vi "GetSpeed.vi"(9 "pulse positions":T2, 10 "channel":T3, 11 "Map":T1) -> (2 "pulse position data":dbl[](array[numeric]), 3 "speed (RPM)":dbl)   [LabVIEW 2017, in "AnalysisHelper.lvlib"]
uses:
  <vilib>/addons/InsightCM/Utilities/Analysis/Shared/AnalysisHelper.lvlib
  <vilib>/addons/InsightCM/Utilities/Analysis/Shared/controls/Channel.ctl
  <vilib>/addons/InsightCM/Utilities/Analysis/Shared/controls/SpeedType.ctl
  <vilib>/addons/InsightCM/Utilities/Analysis/Shared/controls/Feature.ctl
  <vilib>/addons/InsightCM/Utilities/Analysis/Shared/controls/AmplitudeScale.ctl
  <vilib>/addons/InsightCM/Utilities/Analysis/Shared/controls/PulsePositions.ctl
  <vilib>/addons/PointValueMap/controls/PointMap.ctl
  <vilib>/addons/PointValueMap/subVIs/Point_Read_double.vi
  <vilib>/addons/PointValueMap/PointValueMap.lvlib
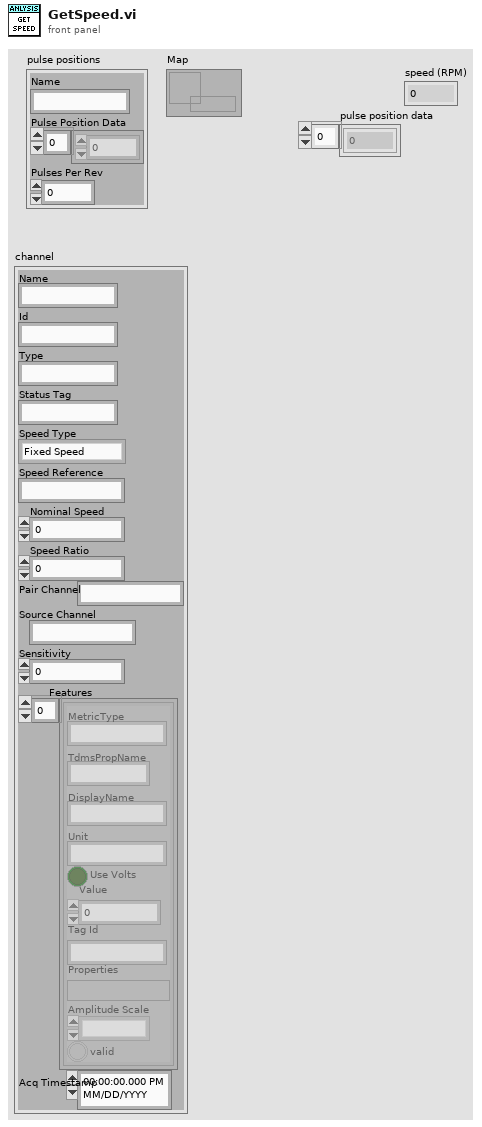
[diagram p1: front panel]
types:
  T1 = typedef "PointValueMap.lvlib/PointMap.ctl" = refnum<data-value>
  T2 = typedef "AnalysisHelper.lvlib/PulsePositions.ctl" = cluster{"Name":string, "Pulse Position Data":dbl[], "Pulses Per Rev":i32}
  T3 = typedef "AnalysisHelper.lvlib/Channel.ctl" = cluster{"Name":string, "Id":string, "Type":string, "Status Tag":string, "Speed Type":T4, "Speed Reference":string, "Nominal Speed":dbl, "Speed Ratio":dbl, "Pair Channel":string, "Source Channel":string, "Sensitivity":dbl, "Features":T5[], "Acq Timestamp":timestamp}
  T4 = typedef "AnalysisHelper.lvlib/SpeedType.ctl" = enum16{"Fixed Speed", "Tachometer", "From Map"}
  T5 = typedef "AnalysisHelper.lvlib/Feature.ctl" = cluster{"MetricType":string, "TdmsPropName":string, "DisplayName":string, "Unit":string, "Use Volts":bool, "Value":dbl, "Tag Id":string, "Properties":variant, "Amplitude Scale":T6, "valid":bool}
  T6 = typedef "AnalysisHelper.lvlib/AmplitudeScale.ctl" = enum16{"rms", "peak", "pk-pk"}
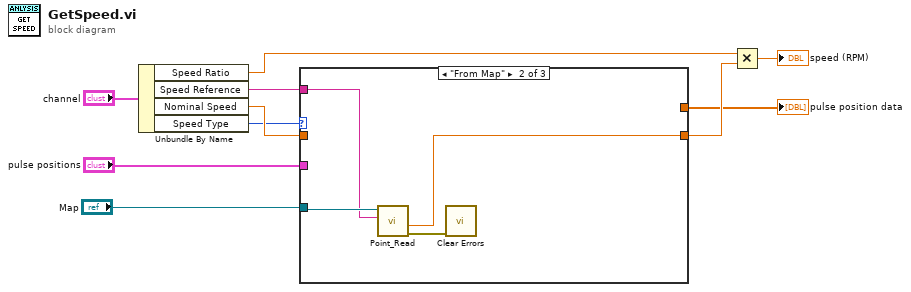
[diagram p0: block diagram]
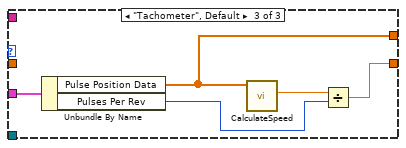
[diagram p3: hidden frame]
diagram:
  n1 = Unbundle By Name("channel") -> ("Speed Ratio"=w5:dbl, "Speed Reference"=w1:string, "Nominal Speed"=w6:dbl, "Speed Type"=w2:T4)
  n2 = case shown="\"From Map\"" w2 {
    tunnel: [w11 w13 w16] -> w7
    tunnel: "pulse positions" -> [_ _ w20]
    tunnel: w6 -> [w11 _ _]
    tunnel: [_ _ w19] -> w4
    tunnel: "Map" -> [_ w15 _]
    tunnel: w1 -> [_ w14 _]
    frame "Fixed Speed" {
    }
    frame "From Map" {
      n3 = call-poly <vilib>:"Point_Read.vi"("Tag"=w14, "Map"=w15) -> ("Error Out"=w12:errorcluster, "Value"=w13:dbl)  [unwired: 4 in, 4 out]
      n4 = call <vilib>:"Clear Errors.vi"("error in (no error)"=w12) -> ()  [unwired: 5 in, 2 out]
    }
    frame "Tachometer", Default {
      n5 = Unbundle By Name(w20) -> ("Pulse Position Data"=w19:dbl[], "Pulses Per Rev"=w17:i32)
      n6 = call <vilib>:"CalculateSpeed.vi"("Pulse Positions"=w19) -> ("Speed (RPM)"=w18:dbl)  [unwired: 9 in, 1 out]
      n7 = Divide(x=w18, y=w17) -> (x/y=w16:dbl)
    }
  }
  "pulse position data" <- w4
  n8 = Multiply(x=w5, y=w7) -> (x*y=→"speed (RPM)":dbl)
